vi "fpga_8ch_MUX-Poller_BaselineCh.vi"(1 "Timestamp bundle":T3, 2 "Data available":T2, 3 "Scheduler":u8, 4 "Baseline CH":u8=8) -> (0 "8Ch Timestamps":T1)   [LabVIEW 2011]
uses:
  Time Stamp Data.ctl
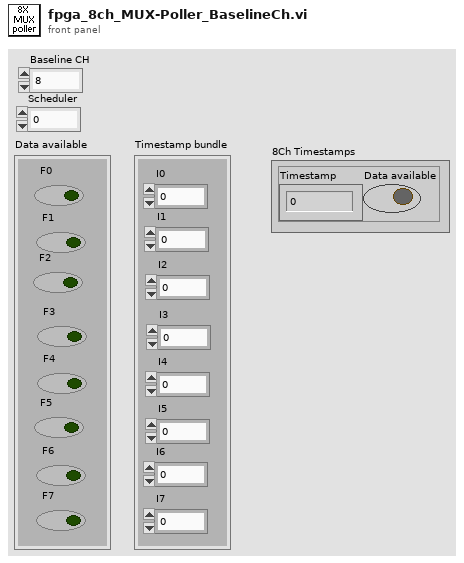
[diagram p1: front panel]
types:
  T1 = typedef "Time Stamp Data.ctl" = cluster{"Timestamp":u32, "Data available":bool}
  T2 = cluster{"F0":bool, "F2":bool, "F3":bool, "F4":bool, "F5":bool, "F6":bool, "F7":bool, "F1":bool}
  T3 = cluster{"I0":u32, "I1":u32, "I2":u32, "I3":u32, "I4":u32, "I5":u32, "I6":u32, "I7":u32}
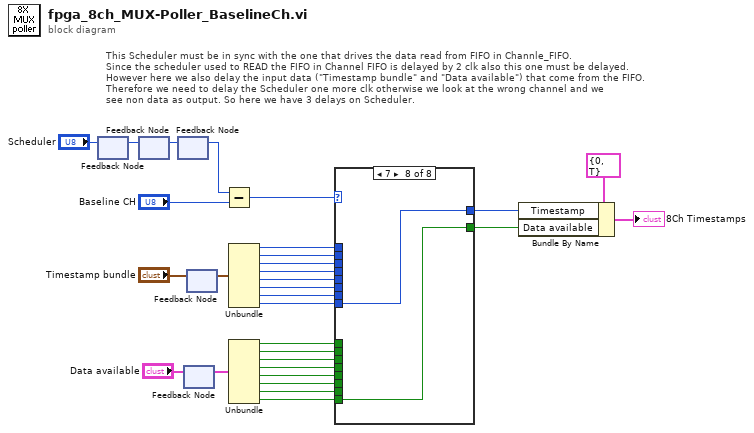
[diagram p0: block diagram]
diagram:
  # "This Scheduler must be in sync with the one that drives the data read from FIFO in Channle_FIFO.\nSince the scheduler used to READ the FIFO in Channel FIFO is delayed by 2 clk also this one must be delayed.\nHowever here we also delay the input data (\"Timestamp bundle\" and \"Data available\") that come from the FIFO.\nTherefore we need to delay the Scheduler one more clk otherwise we look at the wrong channel and we \nsee non data as output. So here we have 3 delays on Scheduler."
  n1 = feedback-in #1("Scheduler") -> ()
  n2 = feedback #1() -> (w4:u8)  [unwired: 1 in]
  n3 = feedback-in #2(w4) -> ()
  n4 = feedback #2() -> (w5:u8)  [unwired: 1 in]
  n5 = feedback #3() -> (w2:u8)  [unwired: 1 in]
  n6 = feedback-in #3(w5) -> ()
  n7 = feedback-in #4("Data available") -> ()
  n8 = feedback #4() -> (w27:T2)  [unwired: 1 in]
  n9 = feedback-in #5("Timestamp bundle") -> ()
  n10 = feedback #5() -> (w28:T3)  [unwired: 1 in]
  n11 = Subtract(x=w2, y="Baseline CH") -> (x-y=w1:u8)
  n12 = Unbundle(w28) -> ("I0"=w23:u32, "I1"=w22:u32, "I2"=w21:u32, "I3"=w20:u32, "I4"=w19:u32, "I5"=w18:u32, "I6"=w17:u32, "I7"=w16:u32)
  n13 = Unbundle(w27) -> ("F0"=w15:bool, "F2"=w14:bool, "F3"=w13:bool, "F4"=w12:bool, "F5"=w11:bool, "F6"=w10:bool, "F7"=w9:bool, "F1"=w8:bool)
  n14 = case shown="7" w1 {
    tunnel: w23 -> [w32 _ _ _ _ _ _ _]
    tunnel: w22 -> [_ w34 _ _ _ _ _ _]
    tunnel: w21 -> [_ _ w36 _ _ _ _ _]
    tunnel: w20 -> [_ _ _ w38 _ _ _ _]
    tunnel: w19 -> [_ _ _ _ w40 _ _ _]
    tunnel: w18 -> [_ _ _ _ _ w42 _ _]
    tunnel: w17 -> [_ _ _ _ _ _ w44 _]
    tunnel: w16 -> [_ _ _ _ _ _ _ w46]
    tunnel: w15 -> [w31 _ _ _ _ _ _ _]
    tunnel: w14 -> [_ w33 _ _ _ _ _ _]
    tunnel: w13 -> [_ _ w35 _ _ _ _ _]
    tunnel: w12 -> [_ _ _ w37 _ _ _ _]
    tunnel: w11 -> [_ _ _ _ w39 _ _ _]
    tunnel: w10 -> [_ _ _ _ _ w41 _ _]
    tunnel: w9 -> [_ _ _ _ _ _ w43 _]
    tunnel: w8 -> [_ _ _ _ _ _ _ w45]
    tunnel: [w32 w34 w36 w38 w40 w42 w44 w46] -> w7
    tunnel: [w31 w33 w35 w37 w39 w41 w43 w45] -> w6
    frame 0, Default {
    }
    frame 1 {
    }
    frame 2 {
    }
    frame 3 {
    }
    frame 4 {
    }
    frame 5 {
    }
    frame 6 {
    }
    frame 7 {
    }
  }
  n15 = Bundle By Name(cluster=T1 {"Timestamp"=0, "Data available"=TRUE} ("8Ch Timestamps"), "Timestamp"=w7, "Data available"=w6) -> (→"8Ch Timestamps":T1)
